vi "LeavePGroupsOut.vi"(6 "Groups":string[][](array[string]), 8 "error in (no error)":errorcluster caption="entrée d'erreur (pas d'erreur)", 9 "y":string[][](array[string]), 10 "X":string[][](array[string]), 11 "LeavePGroupsOut":cluster{"n_groups":i32}={"n_groups"=2}) -> (0 "error out":errorcluster caption="sortie d'erreur", 3 "Split":T1(array[cluster]))   [LabVIEW 2020]
doc: "Leave P Group(s) Out cross-validator\n\nProvides train/test indices to split data according to a third-party provided group. This group information can be used to encode arbitrary domain specific stratifications of the samples as integers.\n\nFor instance the groups could be the year of collection of the samples and thus allow for cross-validation against time-based splits.\n\nThe difference between LeavePGroupsOut and LeaveOneGroupOut is that the former builds the test sets with all the samples assigned to p different values of the groups while the latter uses samples all assigned the same groups.\n\nParameters : \n\n- n_groups : int\nNumber of groups (p) to leave out in the test split.\n\n\n\nMethods : Split\n\n\nGenerate indices to split data into training and test set.\n\nParameters : \n\n- X : array-like of shape (n_samples, n_features)\nTraining data, where n_samples is the number of samples and n_features is the number of features.\n\n- y : array-like of shape (n_samples,), default=None\nThe target variable for supervised learning problems.\n\n- groups : array-like of shape (n_samples,)\nGroup labels for the samples used while splitting the dataset into train/test set.\n\nYields : \n\n- train : ndarray\nThe training set indices for that split.\n\n- test : ndarray\nThe testing set indices for that split."
uses:
  LeavePGroupsOut.lvclass
panel:
  out "LeavePGroupsOut.lvclass":refnum<class "LeavePGroupsOut.lvclass">
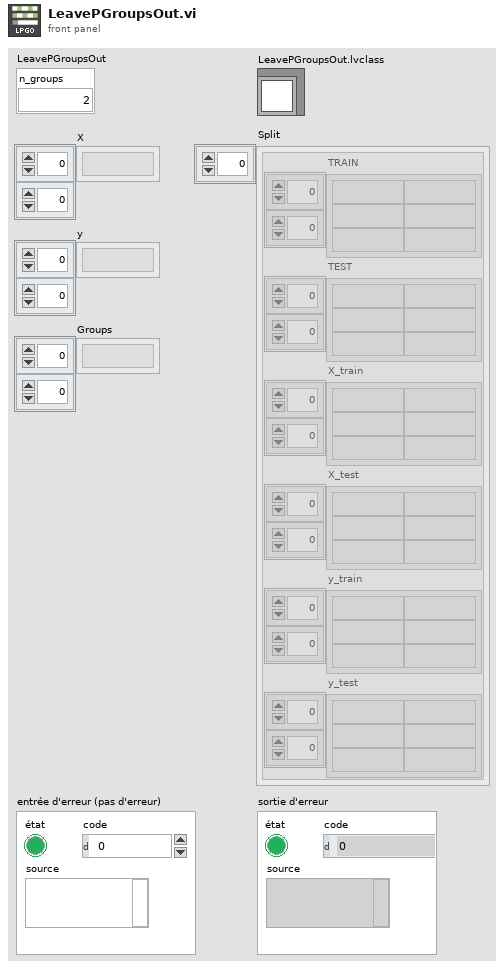
[diagram p1: front panel]
types:
  T1 = cluster{"TRAIN":string[][], "TEST":string[][], "X_train":string[][], "X_test":string[][], "y_train":string[][], "y_test":string[][]}[]
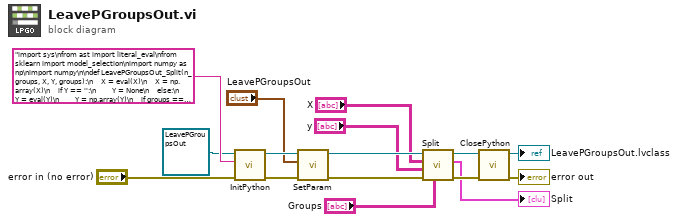
[diagram p0: block diagram]
diagram:
  n1 = call-dynamic "InitPython.vi"("error in (no error)"="error in (no error)", "Python Instruction"="import sys\nfrom ast import literal_eval\nfrom sklearn import model_selection\nimport numpy as np\nimport numpy\n\ndef LeavePGroupsOut_Split(n_groups, X, Y, groups):\n    X = eval(X)\n    X = np.array(X)\n    if Y == '':\n        Y = None\n    else:\n        Y = eval(Y)\n        Y = np.array(Y)\n    if groups == '':\n        groups = None\n    else:\n        groups = eval(groups)\n        groups = np.array(groups)\n    list_return = []\n    try:\n        for train_index, test_index in model_selection.LeavePGroupsOut(n_groups).split(X, Y, groups):\n            list_return = list_return +[\"TRAIN:\", train_index.tolist(), \"TEST:\", test_index.tolist()]\n            X_train, X_test = X[train_index].tolist(), X[test_index].tolist()\n            y_train, y_test = Y[train_index].tolist(), Y[test_index].tolist()\n            list_return = list_return +[\"X_train:\", X_train, \"X_test:\", X_test, \"y_train:\", y_train, \"y_test:\", y_test]\n        return str(list_return)\n    except:\n        erreur = sys.exc_info()\n        typerr = u\"%s\" % (erreur[0])\n        typerr = typerr[typerr.find(\"'\")+1:typerr.rfind(\"'\")]\n        msgerr = u\"%s\" % (erreur[1])\n        message = str('/!\\\\ {0} : {1}'. format(typerr,msgerr))\n        return message", "Scikit-learn en entrée"=refnum<class "LeavePGroupsOut.lvclass"> refnum ("LeavePGroupsOut.lvclass")) -> ("error out"=w14:errorcluster, "Scikit-learn en sortie"=w13:refnum<class "LeavePGroupsOut.lvclass">)  [unwired: 7 in]
  n2 = call-dynamic "SetParam.vi"("error in (no error)"=w14, "LeavePGroupsOut"="LeavePGroupsOut", "LeavePGroupsOut.lvclass"=w13) -> ("error out"=w10:errorcluster, "LeavePGroupsOut.lvclass"=w9:refnum<class "LeavePGroupsOut.lvclass">)  [unwired: 7 in]
  n3 = call-dynamic "Split.vi"("Groups"="Groups", "error in (no error)"=w10, "y"="y", "X"="X", "LeavePGroupsOut.lvclass"=w9) -> ("error out"=w8:errorcluster, "Split"=→"Split":T1, "LeavePGroupsOut.lvclass"=w7:refnum<class "LeavePGroupsOut.lvclass">)  [unwired: 4 in]
  n4 = call-dynamic "ClosePython.vi"("error in (no error)"=w8, "Scikit-learn en entrée"=w7) -> ("error out"=→"error out":errorcluster, "Scikit-learn en sortie"=→"LeavePGroupsOut.lvclass":refnum<class "LeavePGroupsOut.lvclass">)  [unwired: 8 in]
